vi "Save Library.vi"(8 "error in (no error)":errorcluster, 11 "library":refnum<vi>) -> (0 "error out":errorcluster, 3 "library out":refnum<vi>)   [LabVIEW 2020, in "WebServiceImporter.lvlib" / "VI Generator.lvlib"]
uses:
  <vilib>/Platform/WebService/VI Generator/VI Generator.lvlib
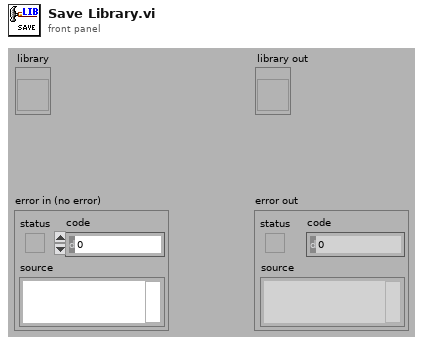
[diagram p1: front panel]
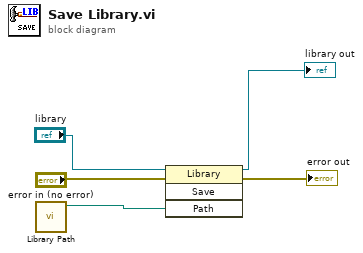
[diagram p0: block diagram]
diagram:
  n1 = call <vilib>:"Library Path.vi"() -> ("Path (out)"=w1:path)  [unwired: 10 in, 1 out]
  n2 = invoke class="Library" method="Save"(reference="library", error in="error in (no error)", "Path"=w1) -> (reference out=→"library out":refnum<vi>, error out=→"error out":errorcluster)  [unwired: 1 in, 2 out]
